vi "Request Task Run Info.vi"(8 "error in (no error)":errorcluster, 10 "Promise":refnum<class "Promise.lvclass">, 11 "VolatusCore in":refnum<class "VolatusCore.lvclass">) -> (0 "error out":errorcluster, 3 "VolatusCore out":refnum<class "VolatusCore.lvclass">)   [LabVIEW 2020, in "Volatus.lvlib" / "VolatusCore.lvclass"]
uses:
  VolatusCore.lvclass
  VolatusCore.lvclass/VolatusCore.ctl
  TaskRunInfoArrayValue/TaskRunInfoArrayValue.lvclass
  lv-promises/Promises/Promise/Promise.lvclass
  C:/dev/lv20CE/relink/lv-promises/Promises/Value/Value.lvclass
  C:/dev/lv20CE/relink/lv-volatus/Volatus/TaskRunInfoArrayValue/TaskRunInfoArrayValue.lvclass
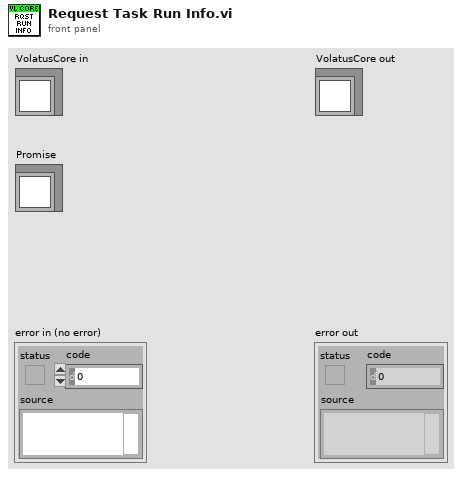
[diagram p1: front panel]
types:
  T1 = typedef "Volatus.lvlib/Task Hierarchy.ctl" = string[]
  T2 = typedef "Volatus.lvlib/Task Run Info.ctl" = cluster{"Hierarchy":T1, "State":T3}
  T3 = typedef "Volatus.lvlib/Task State.ctl" = enum16{"Unknown", "Idle", "Initializing", "Starting", "Running", "Stopping", "Stopped", "Error - Init", "Error - Start", "Error - Run", "Error - Stop"}
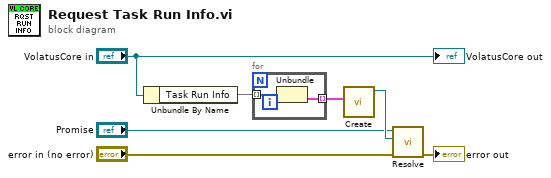
[diagram p0: block diagram]
diagram:
  n1 = Unbundle By Name("VolatusCore in") -> ("Task Run Info"=w6:map{T1, T2})
  n2 = for {
    tunnel: w6 -> [w9] mode=indexing
    tunnel: [w8] -> w5 mode=indexing
    n3 = Unbundle(w9) -> ("Run Info"=w8:T2)  [unwired: 1 out]
  }
  n4 = call "Create.vi"("Task Run Info"=w5) -> ("TaskRunInfoArrayValue out"=w4:refnum<class "TaskRunInfoArrayValue.lvclass">)  [unwired: 10 in]
  n5 = call "Resolve.vi"("error in (no error)"="error in (no error)", "Result"=w4, "Promise in"="Promise") -> ("error out"=→"error out":errorcluster)  [unwired: 7 in, 1 out]
  "VolatusCore out" <- "VolatusCore in"
